vi "Set Acquisition Callback.vi"(8 "error in (no error)":errorcluster, 9 "Camera Status":refnum<vi>, 10 "New Frame Arrival":refnum<vi>, 11 "Camera_Prime95B in":refnum<class "Camera_Prime95B.lvclass">) -> (0 "error out":errorcluster, 3 "Camera_Prime95B out":refnum<class "Camera_Prime95B.lvclass">)   [LabVIEW 2020, in "Camera_Prime95B.lvlib" / "Camera_Prime95B.lvclass"]
uses:
  Camera_Prime95B.lvclass
  Camera_Prime95B.lvclass/Camera_Prime95B.ctl
  E:/Development/DevHardSoftware/MicroscopyFramework/Model/Hardware Layer/Real Hardware/Camera_Prime95B/Camera_Prime95B/Dependencies/PVCamNET.dll
  Dependencies/PVCamNET.dll
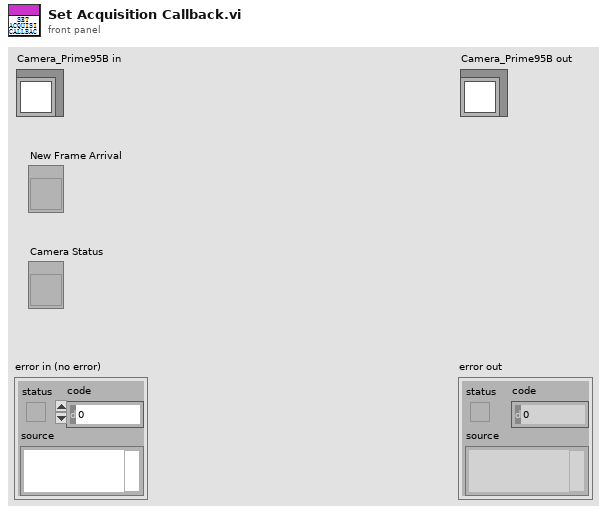
[diagram p1: front panel]
types:
  T1 = typedef "Device.lvlib/DeviceStatus.ctl" = i32
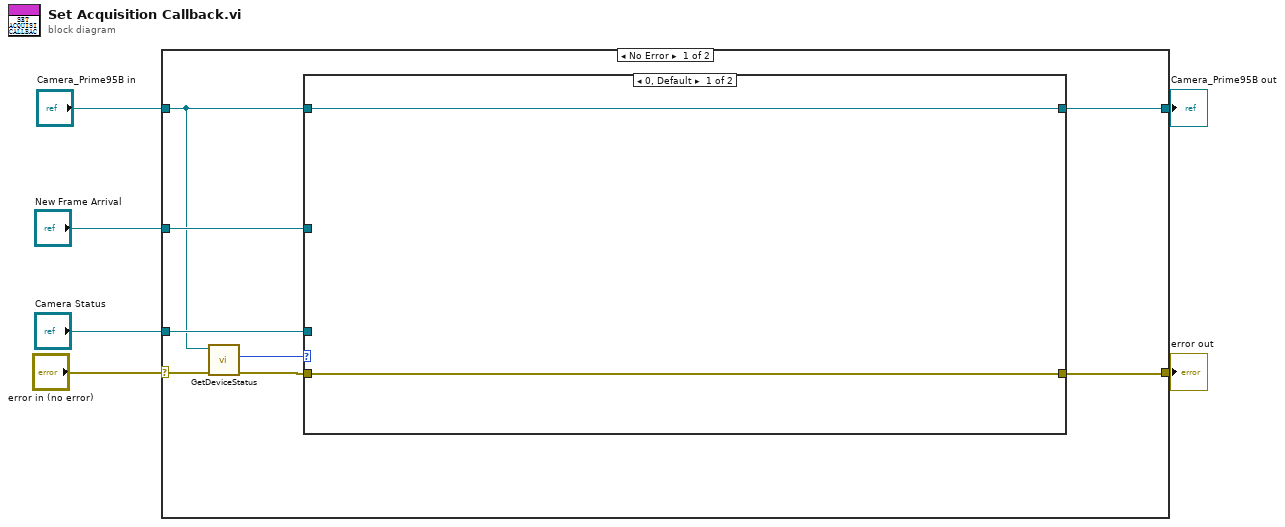
[diagram p0: block diagram]
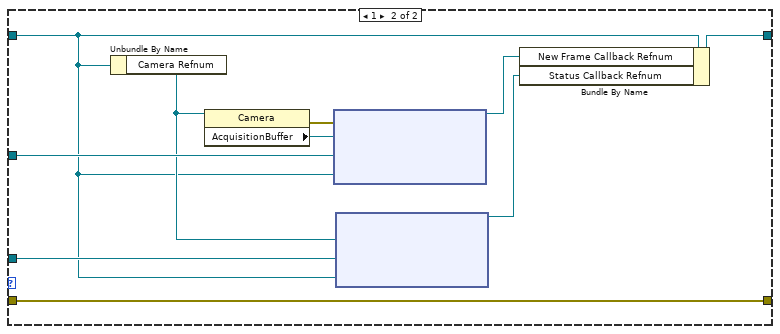
[diagram p2: hidden frame]
diagram:
  n1 = case shown="No Error" "error in (no error)" {
    selector: "error in (no error)" -> [w14 w28]
    tunnel: [w9 w28] -> w5
    tunnel: [w12 w27] -> w3
    tunnel: "Camera_Prime95B in" -> [w8 w27]
    tunnel: "New Frame Arrival" -> [w13 _]
    tunnel: "Camera Status" -> [w11 _]
    frame No Error {
      n2 = call-dynamic "GetDeviceStatus.vi"("error in (no error)"=w14, "Camera_Prime95B in"=w8) -> ("error out"=w10:errorcluster, "Status"=w7:T1)  [unwired: 7 in, 1 out]
      n3 = case shown="0, Default" w7 {
        tunnel: w13 -> [_ w24]
        tunnel: [w15 w23] -> w12
        tunnel: w11 -> [_ w20]
        tunnel: w8 -> [w15 w19]
        tunnel: w10 -> [w16 w17]
        tunnel: [w16 w17] -> w9
        frame 0, Default {
        }
        frame 1 {
          n4 = Unbundle By Name(w19) -> ("Camera Refnum"=w21:refnum<k24>)
          n5 = property class="Camera"(reference=w21) -> (error out=w26:errorcluster, "AcquisitionBuffer"=w25:refnum<k24>)  [unwired: 1 in, 1 out]
          n6 = node(w26, w25, w24, w19) -> (w22:refnum<k27>)  [unwired: 1 in, 1 out]
          n7 = node(w21, w20, w19) -> (w18:refnum<k27>)  [unwired: 2 in, 1 out]
          n8 = Bundle By Name(cluster=w19, "New Frame Callback Refnum"=w22, "Status Callback Refnum"=w18) -> (w23:refnum<class "Camera_Prime95B.lvclass">)
        }
      }
    }
    frame Error {
    }
  }
  "error out" <- w5
  "Camera_Prime95B out" <- w3
